vi "Window-Export timelapse images.vi"(10 "New folder path":path, 11 "Existing AVI path":path) -> ()   [LabVIEW 2013]
uses:
  <vilib>/Utility/miscctls.llb/LVPointTypeDef.ctl
  <vilib>/vision/NI_Vision_Development_Module.lvlib
panel:
  out "Ended":bool
  out "Manually closed":bool
  out "Exporting time-lapse images...":u8(slide) scale=0.0..100.0
  out "# of Frames in exported portion":i32 format="Number of frames: %.0f"
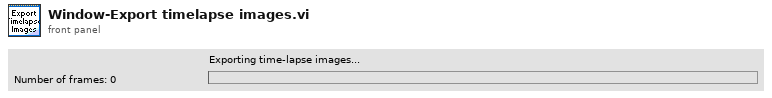
[diagram p1: front panel]
types:
  T1 = typedef "Image Type" = u32
  T2 = typedef "LVPointTypeDef.ctl" = cluster{"Horizontal":i16, "Vertical":i16}
  T3 = typedef "Fixed strings.ctl" = cluster{"ROI file name":string, "Normalised ROI file name":string, "Zplane Pockels values file name":string, "Functional data folder name":string, "Experiment Header file name":string, "Z-stack images folder name":string, "Groups setup rel. path":string, "Groups text file rel. path":string, "TDMS files folder name (F.img)":string, "TDMS files folder name (V.acq)":string, "TDMS files folder name (Pl.acq)":string, "Cycle rel times sequence file":string, "Dynamically called VIs folder name":string, "Time Series folder base name":string}
  T4 = typedef "AVI modes refs cluster.ctl" = cluster{"AVI1 ref":T5, "AVI2 refs":T6[], "AVI # frames":u32[]}
  T5 = typedef "AviRefnum.ctl" = refnum<k1>
  T6 = typedef "IMAQ AVI2 Refnum.ctl" = refnum<k20>
  T7 = typedef "IMAQ Image.ctl" = refnum<image>
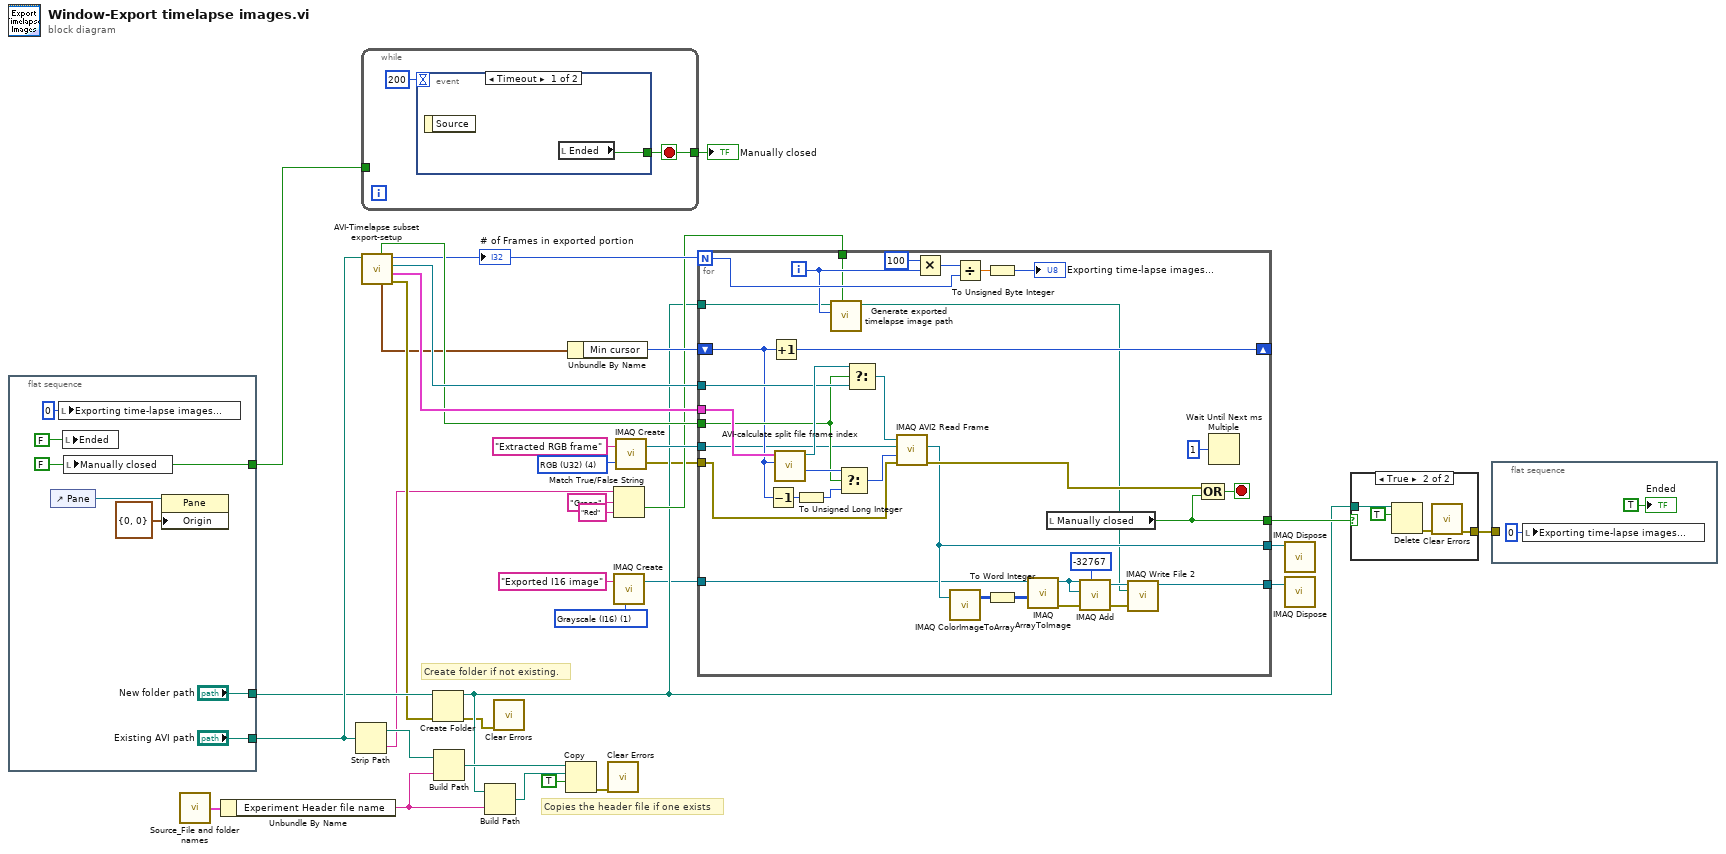
[diagram p0: block diagram]
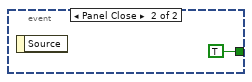
[diagram p3: hidden frame]
diagram:
  w10 = T1 1 items=["Grayscale (U8)", "Grayscale (I16)", "Grayscale (SGL)", "Complex (CSG)", "RGB (U32)", "HSL (U32)", "RGB (U64)", "Grayscale (U16)"] ("Image Type")
  w34 = T1 4 items=["Grayscale (U8)", "Grayscale (I16)", "Grayscale (SGL)", "Complex (CSG)", "RGB (U32)", "HSL (U32)", "RGB (U64)", "Grayscale (U16)"] ("Image Type")
  # "Create folder if not existing."
  # "Copies the header file if one exists"
  n1 = flat-sequence {
    tunnel: ["Existing AVI path"] -> w20
    tunnel: ["New folder path"] -> w19
    tunnel: [w40] -> w6
    frame #0 {
      w40 = FALSE
      n2 = control-ref of="Pane"() -> (w36:refnum<vi>)
      n3 = local write "Exporting time-lapse images..."(u8 0 ("Progress...")) -> ()
      n4 = local write "Ended"(FALSE) -> ()
      n5 = local write "Manually closed"(w40) -> ()
      n6 = property class="Pane"(reference=w36, "Origin"=T2 {"Horizontal"=0, "Vertical"=0}) -> ()  [unwired: 1 in, 2 out]
    }
  }
  n7 = call "Source_File and folder names.vi"() -> ("Fixed strings"=w2:T3)  [unwired: 1 in]
  n8 = Unbundle By Name(w2) -> ("Experiment Header file name"=w1:string)
  n9 = Strip Path(path=w20) -> (stripped path=w26:path, name=w13:string)
  n10 = while {
    tunnel: [w43] -> w35
    tunnel: w6 -> [_]
    stop <- w43 stop-if-true
    n11 = event shown="[0] Timeout" {
      selector: _ -> [_ _]
      dyn-events: _ -> [_ _]
      timeout: 200 -> [_ _]
      tunnel: [w45 TRUE] -> w43
      event Timeout {
        n12 = event-data() -> ()  [unwired: 1 in, 1 out]
        n13 = local read "Ended"() -> (w45:bool)
      }
      event Panel Close {
        n14 = event-data() -> ()  [unwired: 1 in, 1 out]
      }
    }
  }
  "Manually closed" <- w35
  n15 = call "AVI-Timelapse subset export-setup.vi"("AVI path & name"=w20) -> ("error out"=w18:errorcluster, "AVI modes refs"=w32:T4, "AVI Refnum (duplicate)"=w30:T6, "# of Frames in exported portion"=w17:i32, "Extraction cursors"=w16:cluster{"Min cursor":i32, "Max cursor":i32}, "Export all split AVI files as one"=w21:bool)  [unwired: 5 in]
  "# of Frames in exported portion" <- w17
  n16 = Create Folder(path (use dialog)=w19, error in=w18) -> (created path=w11:path, error out=w3:errorcluster)  [unwired: 1 in, 1 out]
  n17 = Build Path(base path=w26, name or relative path=w1) -> (appended path=w25:path)
  n18 = Build Path(base path=w11, name or relative path=w1) -> (appended path=w24:path)
  n19 = call <vilib>:"Clear Errors.vi"("error in (no error)"=w3) -> ()  [unwired: 6 in, 1 out]
  n20 = Copy(9:TRUE ("overwrite (F)"), 10:w24, 11:w25) -> (0:w4:errorcluster)  [unwired: 2 in, 2 out]
  n21 = Unbundle By Name(w16) -> ("Min cursor"=w29:i32)
  n22 = call <vilib>:"Clear Errors.vi"("error in (no error)"=w4) -> ()  [unwired: 6 in, 1 out]
  n23 = Match True/False String(2:"Red" ("false string"), 3:"Green" ("pattern"), 4:w13) -> (0:w12:bool)  [unwired: 1 out]
  n24 = call "IMAQ Create"("Image Name"="Exported I16 image", "Image Type"=w10) -> ("New Image"=w8:T7)  [unwired: 2 in, 2 out]
  n25 = call "IMAQ Create"("Image Name"="Extracted RGB frame", "Image Type"=w34) -> ("New Image"=w31:T7, "error out"=w5:errorcluster)  [unwired: 2 in, 1 out]
  n26 = for {
    N: w17 -> [w70]
    tunnel: w30 -> [w80]
    tunnel: w31 -> [w67]
    tunnel: w32 -> [w82]
    tunnel: w21 -> [w78]
    shift-right: [w68] -> _
    shift-left: w29 -> [w69]
    tunnel: [w60] -> w28
    tunnel: [w62] -> w27
    tunnel: w12 -> [w53]
    tunnel: w11 -> [w52]
    tunnel: w8 -> [w50]
    tunnel: [w49] -> w7
    tunnel: w5 -> [w47]
    i -> [w54]
    stop <- w77 stop-if-true
    n27 = Decrement(x=w69) -> (x-1=w72:i32)
    n28 = Increment(x=w69) -> (x+1=w68:i32)
    n29 = call "AVI-calculate split file frame index.vi"("Frame number (unity-based) in"=w69, "AVI modes refs"=w82) -> ("Index of frame in split file"=w79:u32, "AVI2 split file ref"=w81:T6)  [unwired: 6 in, 2 out]
    n30 = To Unsigned Long Integer(number=w72) -> (unsigned 32bit integer=w71:u32)
    n31 = call "Generate exported timelapse image path.vi"("Green if true"=w53, "FOR loop iteration"=w54, "Folder path"=w52) -> ("File path"=w51:path)  [unwired: 8 in]
    n32 = Select(t=w79, s=w78, f=w71) -> (s? t:f=w65:u32)
    n33 = Select(t=w81, s=w78, f=w80) -> (s? t:f=w66:T6)
    n34 = call "IMAQ AVI2 Read Frame"("error in (no error)"=w47, "Frame Number"=w65, "Image"=w67, "AVI Refnum"=w66) -> ("error out"=w64:errorcluster, "Image Out"=w60:T7)  [unwired: 5 in, 1 out]
    n35 = Multiply(x=100, y=w54) -> (x*y=w75:i32)
    n36 = call "IMAQ ColorImageToArray"("Image"=w60) -> ("Image Pixels (U32)"=w61:u32[][])  [unwired: 2 in, 3 out]
    n37 = Divide(x=w75, y=w70) -> (x/y=w74:dbl)
    n38 = To Unsigned Byte Integer(number=w74) -> (unsigned 8bit integer=→"Exporting time-lapse images...":u8)
    n39 = To Word Integer(number=w61) -> (16bit integer=w55:i16[][])
    n40 = call "IMAQ ArrayToImage"("Image Pixels (I16)"=w55, "Image"=w50) -> ("error out"=w57:errorcluster, "Image Out"=w48:T7)  [unwired: 8 in]
    n41 = local read "Manually closed"() -> (w62:bool)
    n42 = call "IMAQ Add"("Image Src A"=w48, "Constant"=i16 -32767, "Image Dst"=w48, "error in (no error)"=w57) -> ("Image Dst Out"=w59:T7, "error out"=w58:errorcluster)  [unwired: 3 in]
    n43 = call-poly "IMAQ Write File 2"("error in (no error)"=w58, "File Path"=w51, "Image"=w59) -> ("Image Out (duplicate)"=w49:T7)  [unwired: 7 in, 1 out]
    n44 = Compound Arithmetic op=OR(w64, w62) -> (w77:bool)
    n45 = Wait Until Next ms Multiple(millisecond multiple=u32 1) -> ()  [unwired: 1 out]
  }
  n46 = call "IMAQ Dispose"("Image"=w28) -> ()  [unwired: 5 in, 1 out]
  n47 = call "IMAQ Dispose"("Image"=w7) -> ()  [unwired: 5 in, 1 out]
  n48 = case shown="True" w27 {
    tunnel: w11 -> [_ w86]
    tunnel: [_ w83] -> w22
    frame False {
    }
    frame True {
      n49 = Delete(path (use dialog)=w86, entire hierarchy (F)=TRUE) -> (error out=w85:errorcluster)  [unwired: 3 in, 2 out]
      n50 = call <vilib>:"Clear Errors.vi"("error in (no error)"=w85) -> ("error out"=w83:errorcluster)  [unwired: 6 in]
    }
  }
  n51 = flat-sequence {
    tunnel: w22 -> [_]
    frame #0 {
      n52 = local write "Exporting time-lapse images..."(u8 0 ("Progress...")) -> ()
      "Ended" <- TRUE ("Ended")
    }
  }
